vi "Cluster Get Control Value Change.vi"(10 "variant 2":variant, 11 "variant 1":variant) -> (0 "Value":string, 1 "Different":bool, 2 "Index":i32, 3 "control name":string)   [LabVIEW 2020]
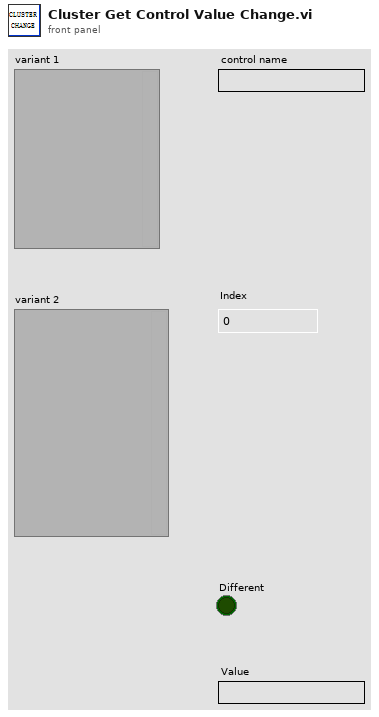
[diagram p1: front panel]
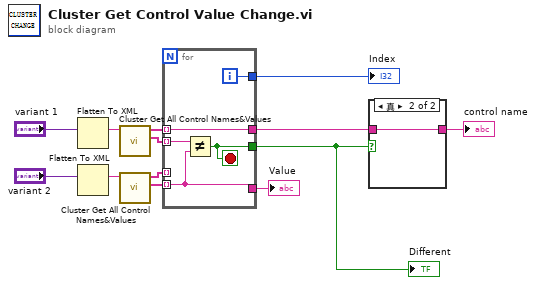
[diagram p0: block diagram]
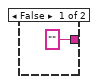
[diagram p2: hidden frame]
diagram:
  n1 = Flatten To XML(6:"variant 1") -> (2:w5:string)
  n2 = Flatten To XML(6:"variant 2") -> (2:w4:string)
  n3 = call "Cluster Get All Control Names&Values.vi"("xml string"=w5) -> ("value"=w11:string[], "name"=w12:string[])  [unwired: 9 in]
  n4 = call "Cluster Get All Control Names&Values.vi"("xml string"=w4) -> ("value"=w10:string[], "name"=w3:string[])  [unwired: 9 in]
  n5 = for {
    tunnel: w12 -> [w17] mode=indexing
    tunnel: w11 -> [w18] mode=indexing
    tunnel: w3 -> [_] mode=indexing
    tunnel: w10 -> [w14] mode=indexing
    tunnel: [w17] -> w6
    tunnel: [w16] -> w7
    tunnel: [w15] -> w2
    tunnel: [w14] -> w1
    i -> [w15]
    stop <- w16 stop-if-true
    n6 = Not Equal?(x=w18, y=w14) -> (x != y?=w16:bool)
  }
  "Index" <- w2
  "Different" <- w7
  "Value" <- w1
  n7 = case shown="真" w7 {
    tunnel: w6 -> [_ w20]
    tunnel: ["" ("Label.Text") w20] -> w13
    frame False {
    }
    frame True {
    }
  }
  "control name" <- w13
